vi "muPathSamplingFPGA28_SkipLiftScheme.vi"() -> ()   [LabVIEW 2017]
uses:
  <vilib>/rvi/Emulation/niFpgaSctlEmulationGetInTimedLoop.vi
  <vilib>/rvi/Emulation/niFpgaProcessEmulError.vi
  <vilib>/rvi/interface/RandomDataEmulation/niFpgaRandomDataHandleErrors.vi
  <vilib>/rvi/Emulation/niFpgaGetClockAttributes.vi
  <vilib>/rvi/Emulation/niFpgaEmulationReportErrorSimple.vi
  <vilib>/rvi/eio/common/nirviEmuTemplateMethod_errors.vi
  <vilib>/rvi/Emulation/niFpgaCriticalErrorInLSC.vi
  <vilib>/rvi/DataTransferAndStorage/Container/XNode/niFpgaContainer.xnode
  <vilib>/rvi/interface/RandomDataEmulation/nirviRandomDataFpgaReadWriteTemplate.vi
  <vilib>/eio/EIONode/EIONode.xnode
panel:
  out "direction_Next":u16
  out "y_image_Next":u16
  out "x_image_Next":u16
  out "Skip threshold":u16
  in  "pixel segment":u32
  out "x output":fxp<+/-,64,29>=0.00029289722442626953
  out "x sensor":fxp<+/-,20,5>
  out "y output":fxp<+/-,64,29>=0.29396580904722214
  out "y sensor":fxp<+/-,20,5>=-0.285125732421875
  in  "XY Clock (uSec)":fxp<+,32,32>=50.0
  out "z output":fxp<+/-,64,29>=-3.5890110712498426
  out "deflection sensor":fxp<+/-,20,5>=-0.271331787109375
  in  "Z Clock (uSec)":fxp<+,32,32>=10.0
  out "ToRead":u32
  in  "Stage Clock (uSec)":fxp<+,32,32>=500.0
  in  "Sampling Clock (uSec)":fxp<+,32,32>=1500.0
  in  "muPathUpdate Clock (uSec)":fxp<+,32,32>=2400.0
  out "zControlMode":bool
  out "a tor buffer":fxp<+,17,1>[](array[numeric])=[1.9999847412109375, 1.9999847412109375, 1.9999847412109375, 1.9999847412109375, 1.9999847412109375, 1.9999847412109375, 1.9999847412109375, 1.9999847412109375, 1.9999847412109375, 1.9999847412109375]
  out "b tor buffer":fxp<+,17,1>[](array[numeric])=[1.9999847412109375, 1.9999847412109375, 1.9999847412109375, 1.9999847412109375, 1.9999847412109375, 1.9999847412109375, 1.9999847412109375, 1.9999847412109375, 1.9999847412109375, 1.9999847412109375]
  out "x_pos":fxp<+/-,50,5>=0.005859375
  out "y_pos":fxp<+/-,50,5>=0.005859375
  out "signalToStop":bool
  in  "deflection control":T1={"SetPoint (V)"=0.0, "scanning I"=0.03125, "scanning P"=0.0498046875, "Initial I (V)"=0.0, "Upper Limit (V)"=8.0, "Lower Limit (V)"=-8.0, "approach I"=0.03125, "approach P"=0.0498046875}
  in  "z control":T2={"SetPoint (V)"=-0.19999980926513672, "I"=0.03125, "P"=0.0498046875, "Initial I (V)"=0.0, "Upper Limit (V)"=8.0, "Lower Limit (V)"=-8.0}
  out "stageIndicator":u8=1
  in  "x threshold":fxp<+/-,20,5>=0.0050048828125
  in  "y threshold":fxp<+/-,20,5>=0.0050048828125
  in  "z threshold":fxp<+/-,20,5>=0.0050048828125
  in  "deflection threshold":fxp<+/-,20,5>=0.0050048828125
  out "length":u16
  out "direction":u16
  out "x_FinalPos":fxp<+/-,50,5>
  out "y_FinalPos":fxp<+/-,50,5>
  out "SettleCheckBuffer":u16=25
  in  "y control":T3={"SetPoint (V)"=0.0, "scanning I"=0.03125, "scanning P"=0.0498046875, "Initial I (V)"=0.0, "Upper Limit (V)"=8.0, "Lower Limit (V)"=-8.0, "move I"=0.03125, "move P"=0.0302734375}
  in  "x control":T3={"SetPoint (V)"=0.0, "scanning I"=0.03125, "scanning P"=0.0498046875, "Initial I (V)"=0.0, "Upper Limit (V)"=8.0, "Lower Limit (V)"=-8.0, "move I"=0.03125, "move P"=0.0498046875}
  out "signalToInitialStageStop":bool
  out "mupathfinishSignal":bool
  in  "ImageToSample":T4={"image size_x"=256, "image size_y"=256, "sample start_x"=0.0, "sample start_y"=0.0, "sample end_x"=3.0, "sample end_y"=3.0}
  out "increment_x":fxp<+/-,50,5>=0.01171875
  out "increment_y":fxp<+/-,50,5>=0.01171875
  out "x_image_pos":u16
  out "y_image_pos":u16
  in  "x_scan threshold":fxp<+/-,20,5>=0.0050048828125
  in  "y_scan threshold":fxp<+/-,20,5>=0.0050048828125
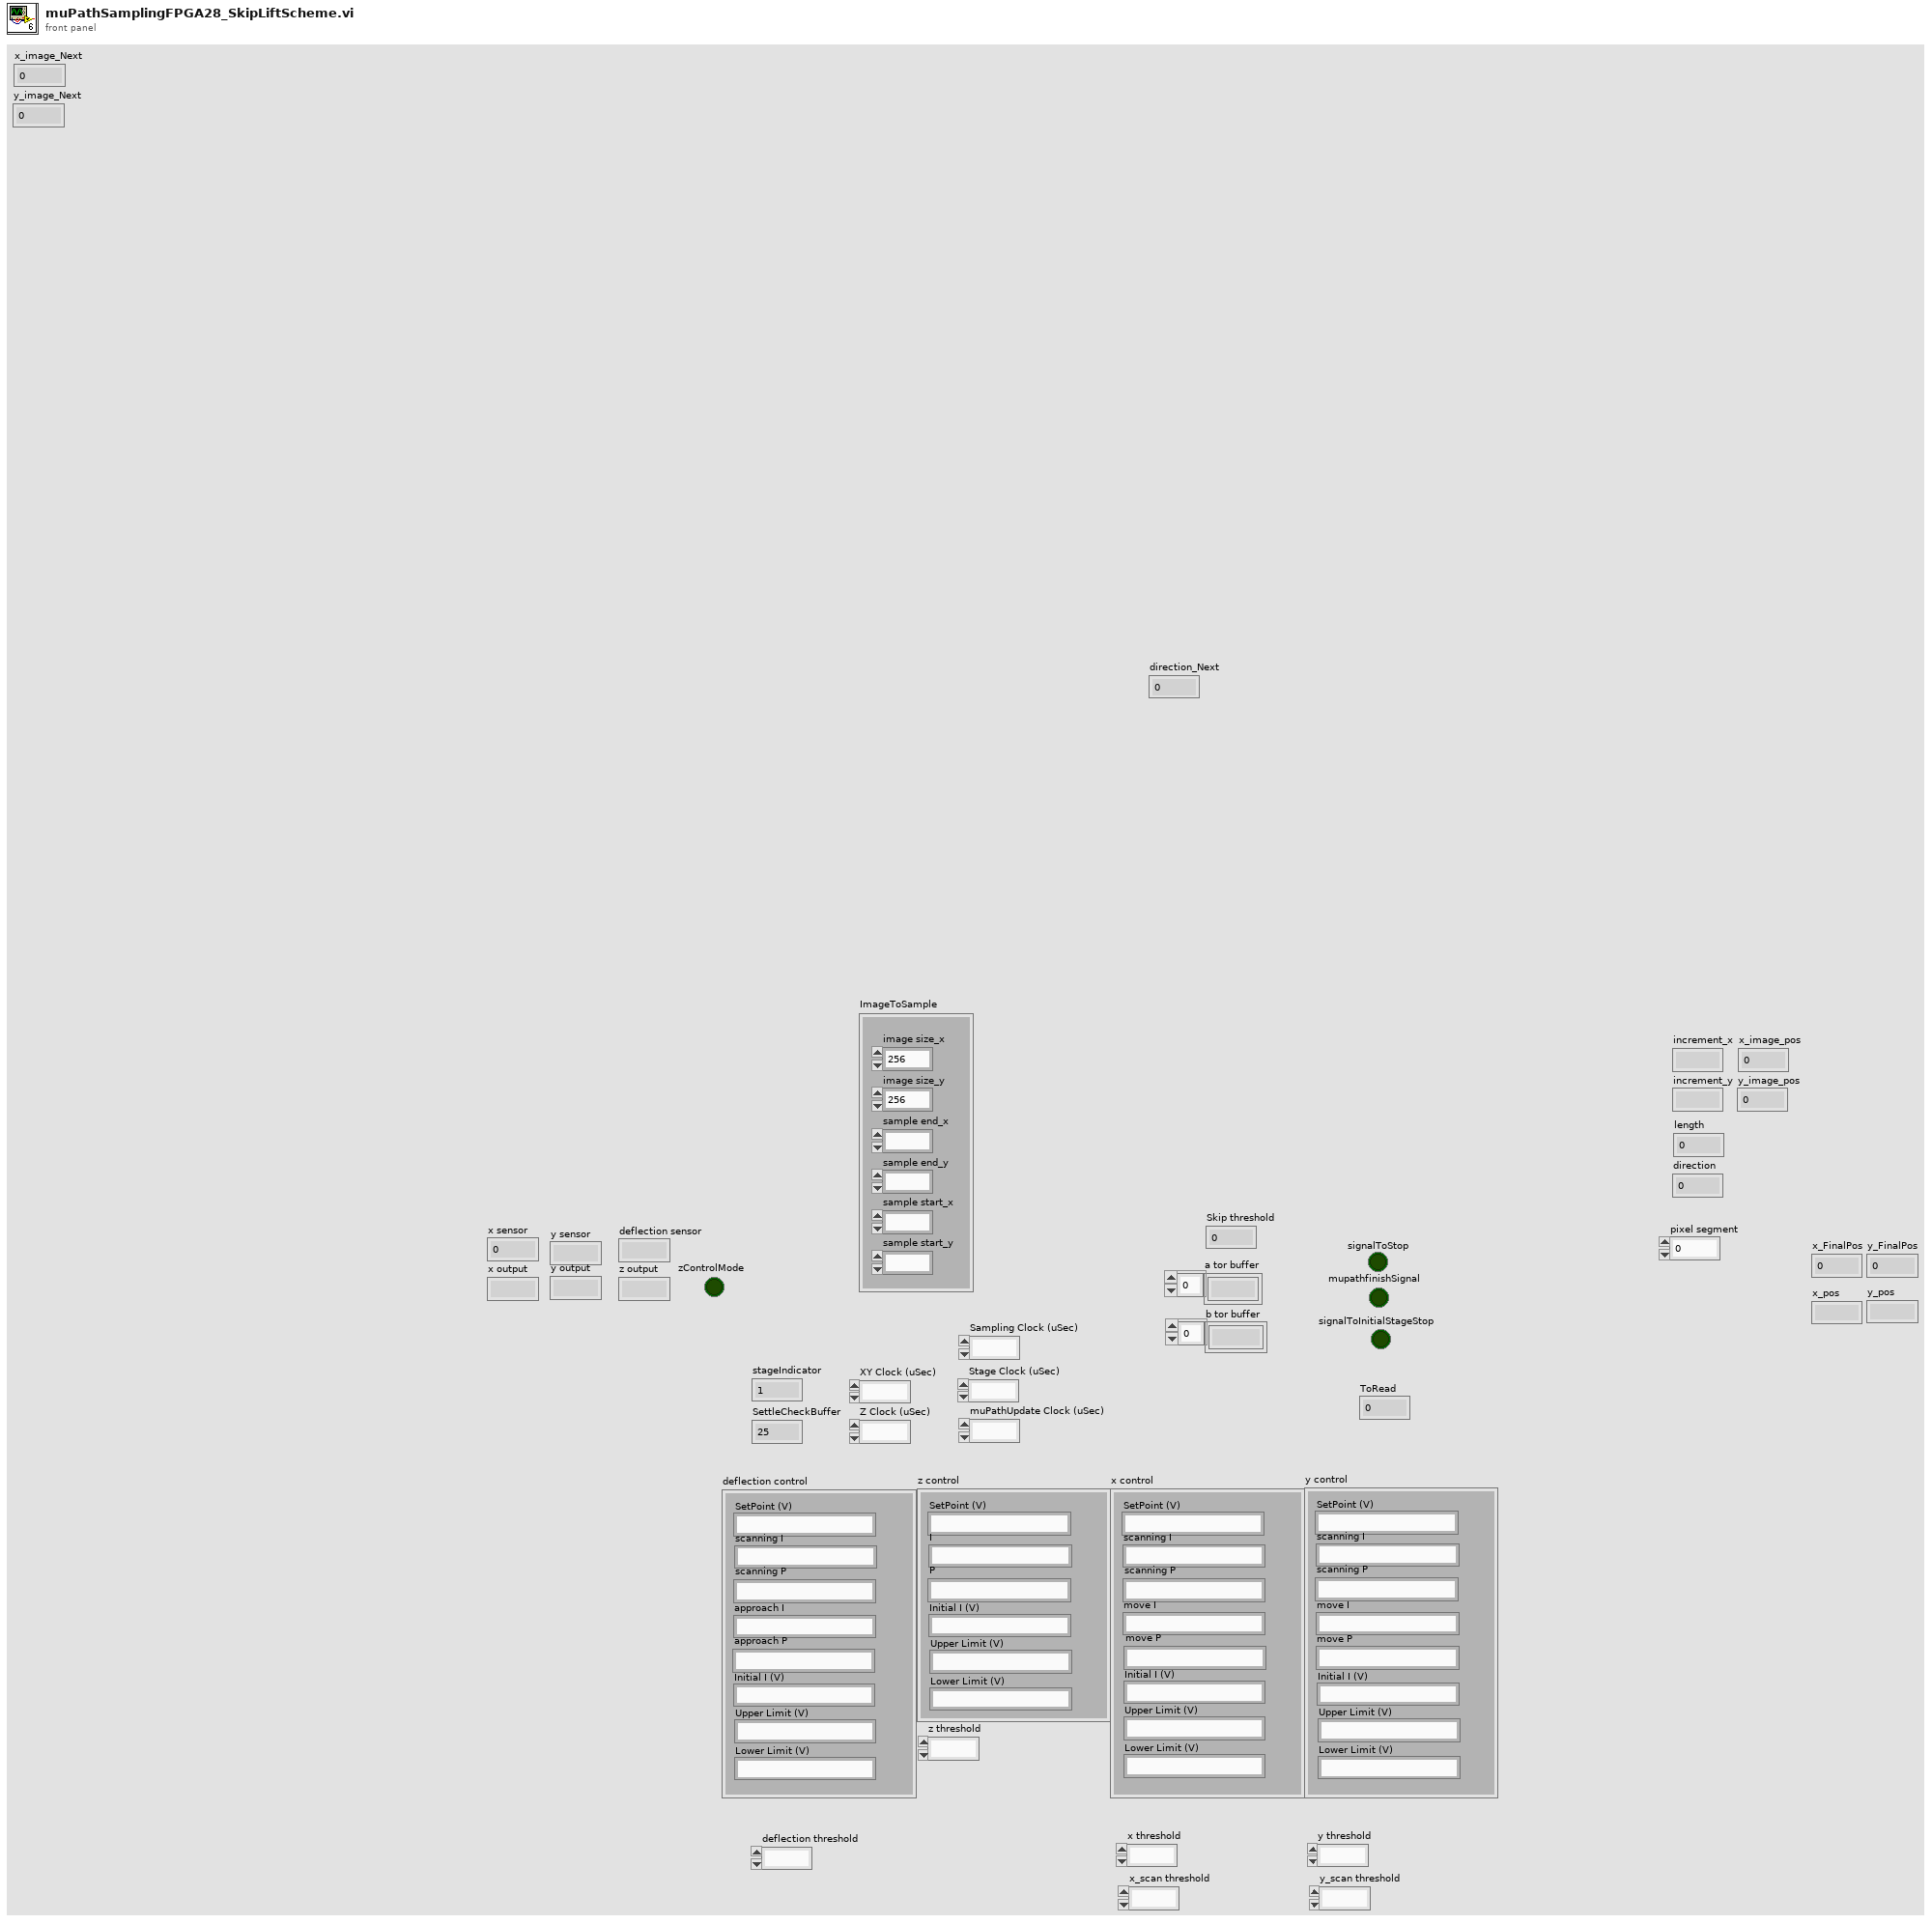
[diagram p1: front panel]
types:
  T1 = cluster{"SetPoint (V)":fxp<+/-,26,5>, "scanning I":fxp<+,21,13>, "scanning P":fxp<+,15,5>, "Initial I (V)":fxp<+/-,10,5>, "Upper Limit (V)":fxp<+/-,26,5>, "Lower Limit (V)":fxp<+/-,26,5>, "approach I":fxp<+,21,13>, "approach P":fxp<+,15,5>}
  T2 = cluster{"SetPoint (V)":fxp<+/-,26,5>, "I":fxp<+,21,13>, "P":fxp<+,15,5>, "Initial I (V)":fxp<+/-,10,5>, "Upper Limit (V)":fxp<+/-,26,5>, "Lower Limit (V)":fxp<+/-,26,5>}
  T3 = cluster{"SetPoint (V)":fxp<+/-,26,5>, "scanning I":fxp<+,21,13>, "scanning P":fxp<+,15,5>, "Initial I (V)":fxp<+/-,10,5>, "Upper Limit (V)":fxp<+/-,26,5>, "Lower Limit (V)":fxp<+/-,26,5>, "move I":fxp<+,21,13>, "move P":fxp<+,15,5>}
  T4 = cluster{"image size_x":u16, "image size_y":u16, "sample start_x":fxp<+/-,26,5>, "sample start_y":fxp<+/-,26,5>, "sample end_x":fxp<+/-,26,5>, "sample end_y":fxp<+/-,26,5>}
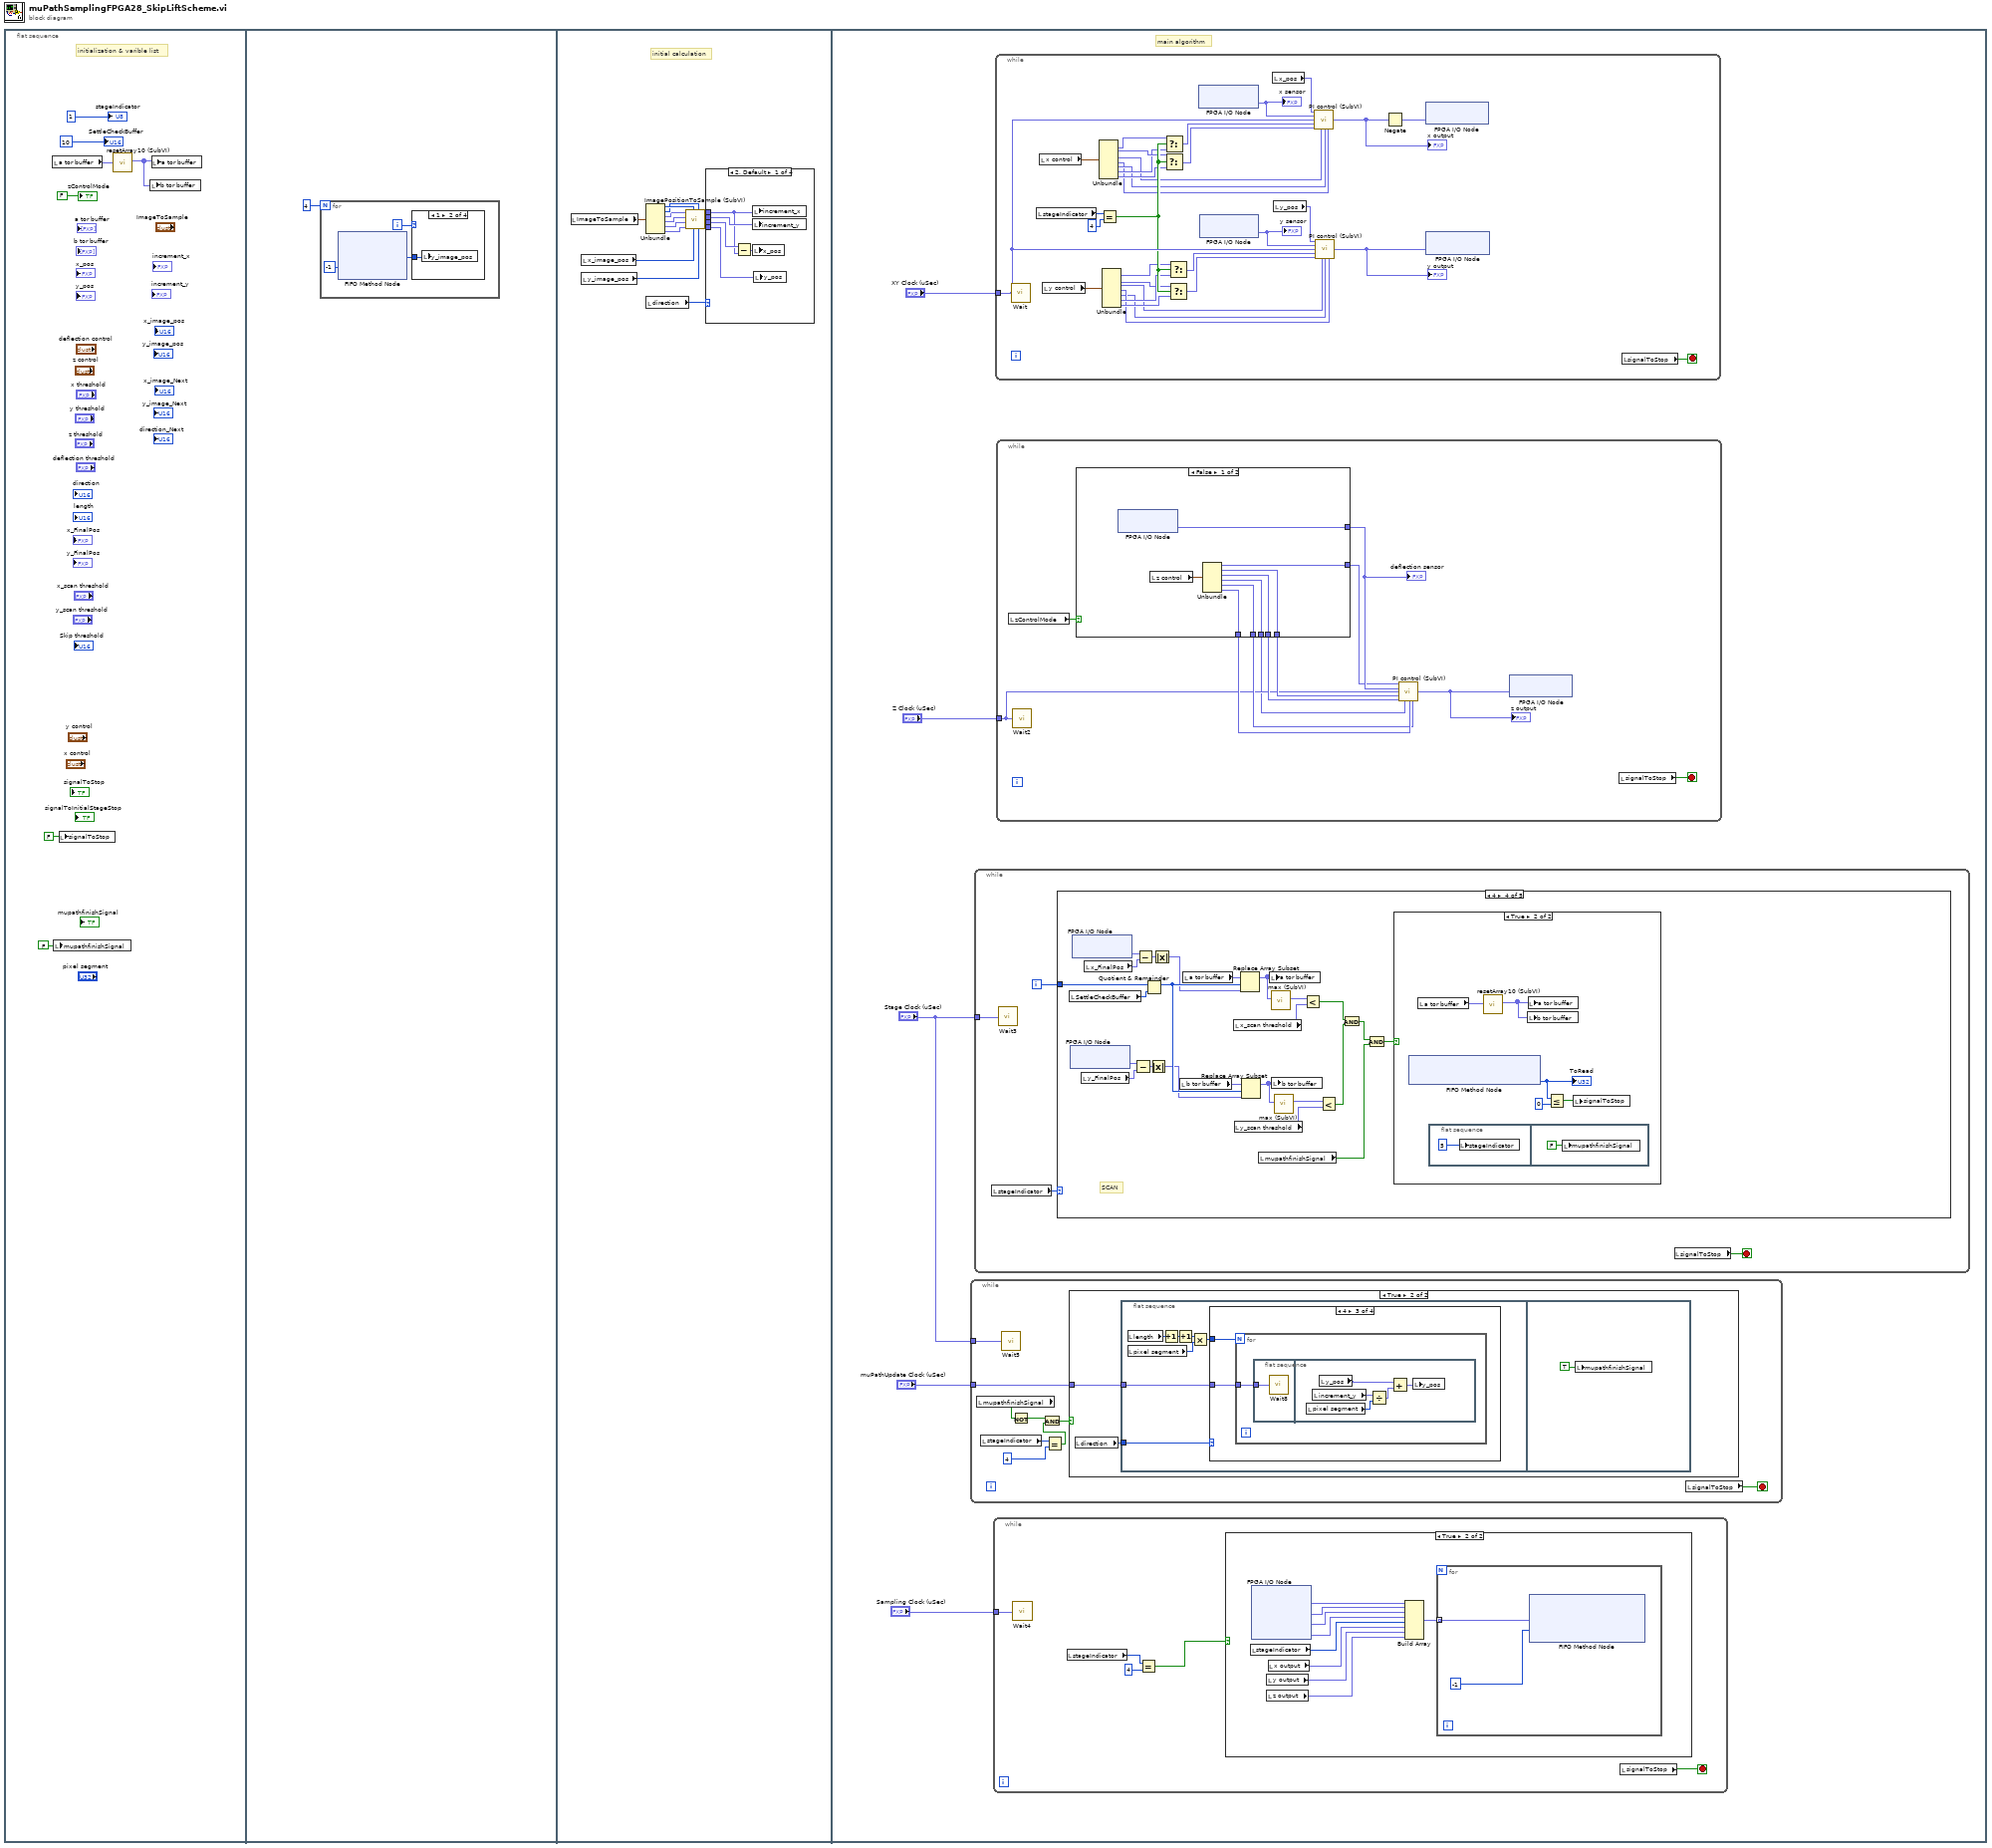
[diagram p0: block diagram]
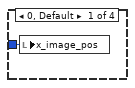
[diagram p2: hidden frame]
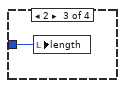
[diagram p3: hidden frame]
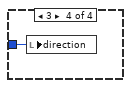
[diagram p4: hidden frame]
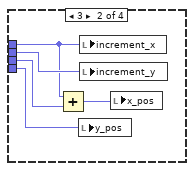
[diagram p5: hidden frame]
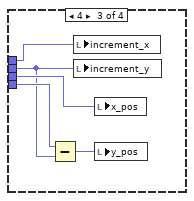
[diagram p6: hidden frame]
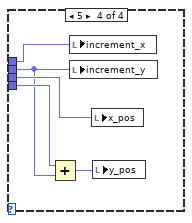
[diagram p7: hidden frame]
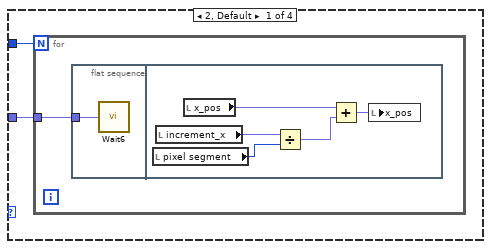
[diagram p9: hidden frame]
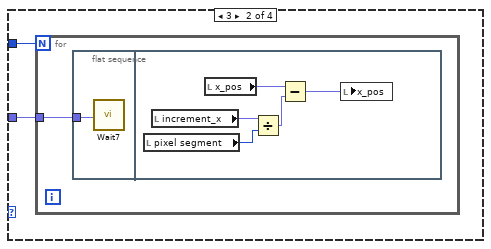
[diagram p10: hidden frame]
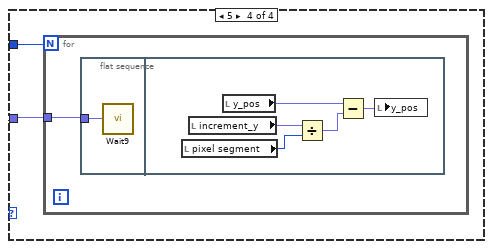
[diagram p11: hidden frame]
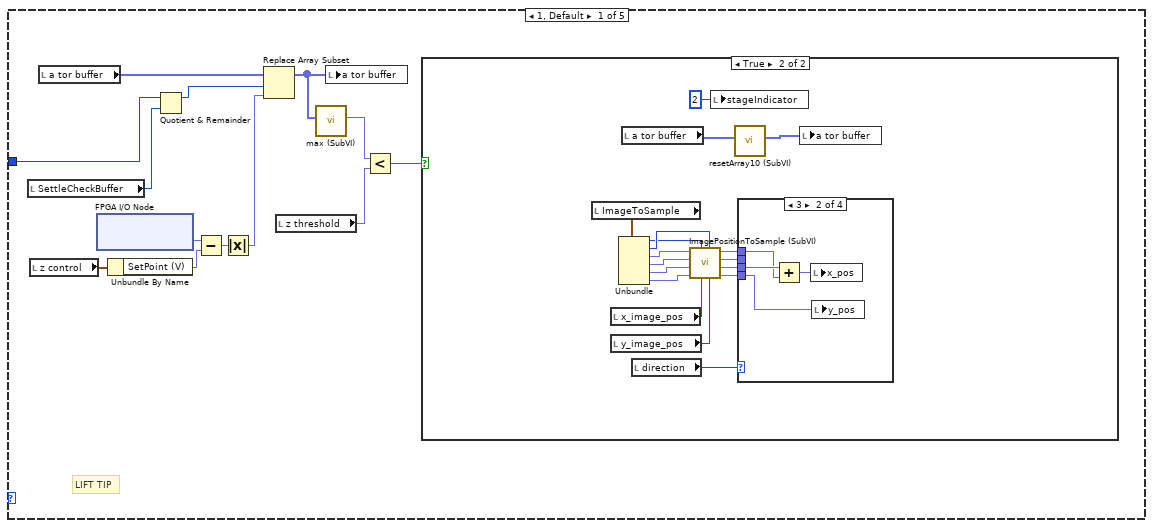
[diagram p13: hidden frame]
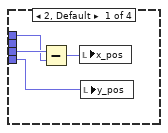
[diagram p15: hidden frame]
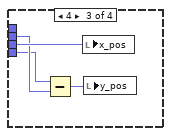
[diagram p16: hidden frame]
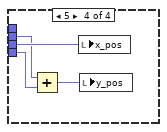
[diagram p17: hidden frame]
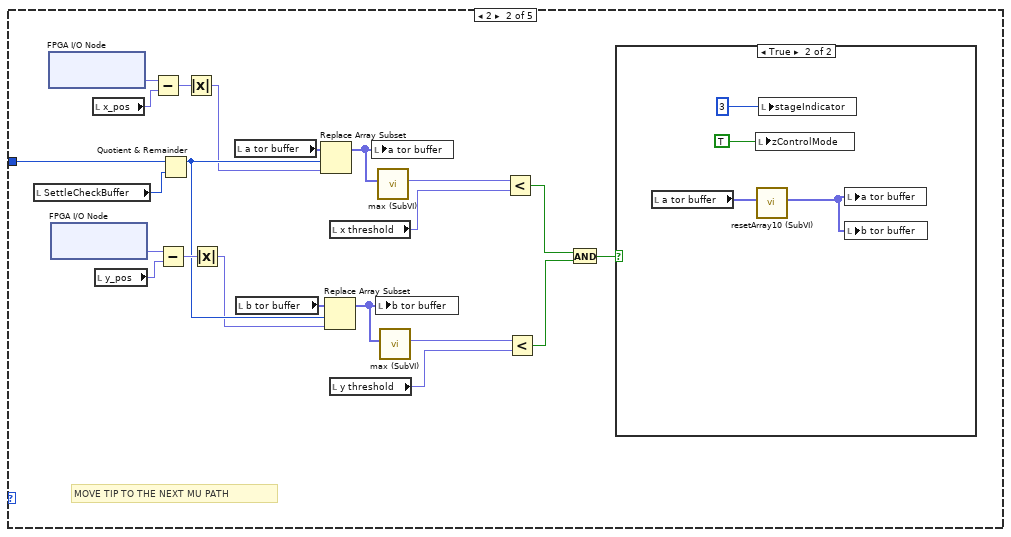
[diagram p18: hidden frame]
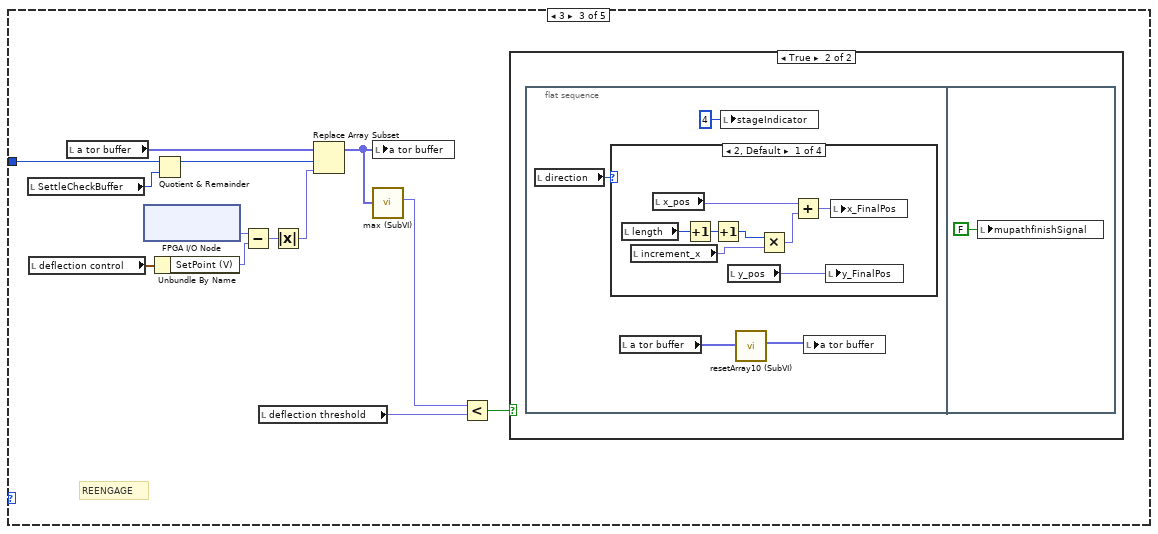
[diagram p20: hidden frame]
diagram:
  n1 = flat-sequence {
    frame #0 {
      # "initialization & varible list"
      n2 = local read "a tor buffer"() -> (w2:fxp<+,17,1>[])
      n3 = local write "mupathfinishSignal"(FALSE ("mupathfinishSignal")) -> ()
      n4 = local write "signalToStop"(FALSE ("signalToStop")) -> ()
      n5 = call "resetArray10 (SubVI).vi"("a samples in"=w2) -> ("a samples out"=w1:fxp<+/-,64,32>[])  [unwired: 10 in]
      n6 = local write "b tor buffer"(w1) -> ()
      n7 = local write "a tor buffer"(w1) -> ()
      "zControlMode" <- FALSE ("zControlMode")
      "stageIndicator" <- u8 1 ("stageIndicator")
      "SettleCheckBuffer" <- u16 10 ("SettleCheckLen")
    }
    frame #1 {
      n8 = for {
        N: 4 -> [_]
        i -> [w11]
        n9 = xnode ("FIFO Method Node")("Timeout"=-1) -> ("Element"=w9:u16)  [unwired: 1 in, 2 out]
        n10 = case shown="1" w11 {
          tunnel: w9 -> [w12 w13 w14 w15]
          frame 0, Default {
            n11 = local write "x_image_pos"(w12) -> ()
          }
          frame 1 {
            n12 = local write "y_image_pos"(w13) -> ()
          }
          frame 2 {
            n13 = local write "length"(w14) -> ()
          }
          frame 3 {
            n14 = local write "direction"(w15) -> ()
          }
        }
      }
    }
    frame #2 {
      # "initial calculation"
      n15 = local read "ImageToSample"() -> (w29:T4)
      n16 = local read "x_image_pos"() -> (w18:u16)
      n17 = local read "y_image_pos"() -> (w17:u16)
      n18 = Unbundle(w29) -> ("image size_x"=w28:u16, "image size_y"=w27:u16, "sample start_x"=w26:fxp<+/-,26,5>, "sample start_y"=w25:fxp<+/-,26,5>, "sample end_x"=w24:fxp<+/-,26,5>, "sample end_y"=w23:fxp<+/-,26,5>)
      n19 = local read "direction"() -> (w16:u16)
      n20 = call "ImagePositionToSample (SubVI).vi"("image_y"=w17, "image size_y"=w27, "image_x"=w18, "image size_x"=w28, "sample end_y"=w23, "sample end_x"=w24, "sample start_y"=w25, "sample start_x"=w26) -> ("sample_y"=w19:fxp<+/-,26,5>, "sample_x"=w20:fxp<+/-,26,5>, "increment_y"=w21:fxp<+/-,26,5>, "increment_x"=w22:fxp<+/-,26,5>)
      n21 = case shown="2, Default" w16 {
        tunnel: w22 -> [w32 w35 w44 w49]
        tunnel: w21 -> [w34 w39 w40 w45]
        tunnel: w20 -> [w33 w36 w42 w47]
        tunnel: w19 -> [w30 w38 w41 w46]
        frame 2, Default {
          n22 = Subtract(x=w33, y=w32) -> (x-y=w31:fxp<+/-,27,6>)
          n23 = local write "increment_y"(w34) -> ()
          n24 = local write "increment_x"(w32) -> ()
          n25 = local write "x_pos"(w31) -> ()
          n26 = local write "y_pos"(w30) -> ()
        }
        frame 3 {
          n27 = Add(x=w35, y=w36) -> (x+y=w37:fxp<+/-,27,6>)
          n28 = local write "y_pos"(w38) -> ()
          n29 = local write "increment_x"(w35) -> ()
          n30 = local write "increment_y"(w39) -> ()
          n31 = local write "x_pos"(w37) -> ()
        }
        frame 4 {
          n32 = Subtract(x=w41, y=w40) -> (x-y=w43:fxp<+/-,27,6>)
          n33 = local write "increment_x"(w44) -> ()
          n34 = local write "increment_y"(w40) -> ()
          n35 = local write "x_pos"(w42) -> ()
          n36 = local write "y_pos"(w43) -> ()
        }
        frame 5 {
          n37 = Add(x=w46, y=w45) -> (x+y=w48:fxp<+/-,27,6>)
          n38 = local write "increment_x"(w49) -> ()
          n39 = local write "increment_y"(w45) -> ()
          n40 = local write "x_pos"(w47) -> ()
          n41 = local write "y_pos"(w48) -> ()
        }
      }
    }
    frame #3 {
      # "main algorithm"
      n42 = while {
        tunnel: "Stage Clock (uSec)" -> [w62]
        tunnel: "muPathUpdate Clock (uSec)" -> [w59]
        stop <- w63 stop-if-true
        n43 = local read "mupathfinishSignal"() -> (w56:bool)
        n44 = local read "stageIndicator"() -> (w61:u8)
        n45 = call "Wait5"("Count(uSec)"=w62) -> ()  [unwired: 1 out]
        n46 = Not(x=w56) -> (.not. x?=w55:bool)
        n47 = Equal?(x=w61, y=u8 4) -> (x = y?=w58:bool)
        n48 = And(x=w55, y=w58) -> (x .and. y?=w57:bool)
        n49 = case shown="True" w57 {
          tunnel: w59 -> [_ w65]
          frame False {
          }
          frame True {
            n50 = local read "direction"() -> (w64:u16)
            n51 = flat-sequence {
              tunnel: w65 -> [w72]
              tunnel: w64 -> [w71]
              frame #0 {
                n52 = local read "length"() -> (w70:u16)
                n53 = local read "pixel segment"() -> (w68:u32)
                n54 = Increment(x=w70) -> (x+1=w67:u16)
                n55 = Increment(x=w67) -> (x+1=w66:u16)
                n56 = Multiply(x=w66, y=w68) -> (x*y=w69:u32)
                n57 = case shown="4" w71 {
                  tunnel: w72 -> [w74 w83 w92 w101]
                  tunnel: w69 -> [w73 w82 w91 w100]
                  frame 2, Default {
                    n58 = for {
                      N: w73 -> [_]
                      tunnel: w74 -> [w75]
                      n59 = flat-sequence {
                        tunnel: w75 -> [w76]
                        frame #0 {
                          n60 = call "Wait6"("Count(uSec)"=w76) -> ()  [unwired: 1 out]
                        }
                        frame #1 {
                          n61 = local read "pixel segment"() -> (w77:u32)
                          n62 = local read "increment_x"() -> (w79:fxp<+/-,50,5>)
                          n63 = local read "x_pos"() -> (w81:fxp<+/-,50,5>)
                          n64 = Divide(x=w79, y=w77) -> (x/y=w78:fxp<+/-,64,5>)
                          n65 = Add(x=w81, y=w78) -> (x+y=w80:fxp<+/-,64,6>)
                          n66 = local write "x_pos"(w80) -> ()
                        }
                      }
                    }
                  }
                  frame 3 {
                    n67 = for {
                      N: w82 -> [_]
                      tunnel: w83 -> [w84]
                      n68 = flat-sequence {
                        tunnel: w84 -> [w85]
                        frame #0 {
                          n69 = call "Wait7"("Count(uSec)"=w85) -> ()  [unwired: 1 out]
                        }
                        frame #1 {
                          n70 = local read "pixel segment"() -> (w86:u32)
                          n71 = local read "increment_x"() -> (w88:fxp<+/-,50,5>)
                          n72 = local read "x_pos"() -> (w90:fxp<+/-,50,5>)
                          n73 = Divide(x=w88, y=w86) -> (x/y=w87:fxp<+/-,64,5>)
                          n74 = Subtract(x=w90, y=w87) -> (x-y=w89:fxp<+/-,64,6>)
                          n75 = local write "x_pos"(w89) -> ()
                        }
                      }
                    }
                  }
                  frame 4 {
                    n76 = for {
                      N: w91 -> [_]
                      tunnel: w92 -> [w93]
                      n77 = flat-sequence {
                        tunnel: w93 -> [w94]
                        frame #0 {
                          n78 = call "Wait8"("Count(uSec)"=w94) -> ()  [unwired: 1 out]
                        }
                        frame #1 {
                          n79 = local read "pixel segment"() -> (w95:u32)
                          n80 = local read "increment_y"() -> (w97:fxp<+/-,50,5>)
                          n81 = local read "y_pos"() -> (w99:fxp<+/-,50,5>)
                          n82 = Divide(x=w97, y=w95) -> (x/y=w96:fxp<+/-,64,5>)
                          n83 = Add(x=w99, y=w96) -> (x+y=w98:fxp<+/-,64,6>)
                          n84 = local write "y_pos"(w98) -> ()
                        }
                      }
                    }
                  }
                  frame 5 {
                    n85 = for {
                      N: w100 -> [_]
                      tunnel: w101 -> [w102]
                      n86 = flat-sequence {
                        tunnel: w102 -> [w103]
                        frame #0 {
                          n87 = call "Wait9"("Count(uSec)"=w103) -> ()  [unwired: 1 out]
                        }
                        frame #1 {
                          n88 = local read "pixel segment"() -> (w105:u32)
                          n89 = local read "increment_y"() -> (w106:fxp<+/-,50,5>)
                          n90 = local read "y_pos"() -> (w108:fxp<+/-,50,5>)
                          n91 = Divide(x=w106, y=w105) -> (x/y=w104:fxp<+/-,64,5>)
                          n92 = Subtract(x=w108, y=w104) -> (x-y=w107:fxp<+/-,64,6>)
                          n93 = local write "y_pos"(w107) -> ()
                        }
                      }
                    }
                  }
                }
              }
              frame #1 {
                n94 = local write "mupathfinishSignal"(TRUE ("mupathfinishSignal")) -> ()
              }
            }
          }
        }
        n95 = local read "signalToStop"() -> (w63:bool)
      }
      n96 = while {
        tunnel: "Stage Clock (uSec)" -> [w127]
        i -> [w126]
        stop <- w129 stop-if-true
        n97 = local read "stageIndicator"() -> (w128:u8)
        n98 = call "Wait3"("Count(uSec)"=w127) -> ()  [unwired: 1 out]
        n99 = case shown="4" w128 {
          tunnel: w126 -> [w141 w190 w210 w269 _]
          frame 1, Default {
            # "LIFT TIP"
            n100 = local read "SettleCheckBuffer"() -> (w140:u16)
            n101 = local read "z control"() -> (w136:T2)
            n102 = local read "a tor buffer"() -> (w139:fxp<+,17,1>[])
            n103 = xnode "FPGA I/O Node"() -> ("Mod1/AI2"=w137:fxp<+/-,20,5>)  [unwired: 1 in, 1 out]
            n104 = Unbundle By Name(w136) -> ("SetPoint (V)"=w135:fxp<+/-,26,5>)
            n105 = Quotient & Remainder(x=w141, y=w140) -> (x-y*floor(x/y)=w134:i32)  [unwired: 1 out]
            n106 = Subtract(x=w137, y=w135) -> (x-y=w138:fxp<+/-,27,6>)
            n107 = Absolute Value(x=w138) -> (abs(x)=w133:fxp<+,26,5>)
            n108 = Replace Array Subset(array=w139, new element=w133, index=w134) -> (w131:fxp<+,17,1>[])
            n109 = local read "z threshold"() -> (w132:fxp<+/-,20,5>)
            n110 = call "max (SubVI).vi"("initialized array"=w131) -> ("y"=w130:fxp<+/-,64,32>)  [unwired: 10 in]
            n111 = local write "a tor buffer"(w131) -> ()
            n112 = Less?(x=w130, y=w132) -> (x < y?=w142:bool)
            n113 = case shown="True" w142 {
              frame False {
              }
              frame True {
                n114 = local read "ImageToSample"() -> (w145:T4)
                n115 = local read "x_image_pos"() -> (w152:u16)
                n116 = local read "y_image_pos"() -> (w153:u16)
                n117 = Unbundle(w145) -> ("image size_x"=w146:u16, "image size_y"=w147:u16, "sample start_x"=w148:fxp<+/-,26,5>, "sample start_y"=w149:fxp<+/-,26,5>, "sample end_x"=w150:fxp<+/-,26,5>, "sample end_y"=w151:fxp<+/-,26,5>)
                n118 = local read "a tor buffer"() -> (w143:fxp<+,17,1>[])
                n119 = local read "direction"() -> (w154:u16)
                n120 = call "ImagePositionToSample (SubVI).vi"("image_y"=w153, "image size_y"=w147, "image_x"=w152, "image size_x"=w146, "sample end_y"=w151, "sample end_x"=w150, "sample start_y"=w149, "sample start_x"=w148) -> ("sample_y"=w155:fxp<+/-,26,5>, "sample_x"=w156:fxp<+/-,26,5>, "increment_y"=w158:fxp<+/-,26,5>, "increment_x"=w157:fxp<+/-,26,5>)
                n121 = local write "stageIndicator"(u8 2 ("stageIndicator")) -> ()
                n122 = call "resetArray10 (SubVI).vi"("a samples in"=w143) -> ("a samples out"=w144:fxp<+/-,64,32>[])  [unwired: 10 in]
                n123 = case shown="3" w154 {
                  tunnel: w155 -> [w163 w167 w168 w173]
                  tunnel: w156 -> [w162 w166 w171 w175]
                  tunnel: w157 -> [w161 w165 _ _]
                  tunnel: w158 -> [_ _ w169 w174]
                  frame 2, Default {
                    n124 = Subtract(x=w162, y=w161) -> (x-y=w160:fxp<+/-,27,6>)
                    n125 = local write "x_pos"(w160) -> ()
                    n126 = local write "y_pos"(w163) -> ()
                  }
                  frame 3 {
                    n127 = Add(x=w166, y=w165) -> (x+y=w164:fxp<+/-,27,6>)
                    n128 = local write "x_pos"(w164) -> ()
                    n129 = local write "y_pos"(w167) -> ()
                  }
                  frame 4 {
                    n130 = Subtract(x=w168, y=w169) -> (x-y=w170:fxp<+/-,27,6>)
                    n131 = local write "x_pos"(w171) -> ()
                    n132 = local write "y_pos"(w170) -> ()
                  }
                  frame 5 {
                    n133 = Add(x=w174, y=w173) -> (x+y=w172:fxp<+/-,27,6>)
                    n134 = local write "x_pos"(w175) -> ()
                    n135 = local write "y_pos"(w172) -> ()
                  }
                }
                n136 = local write "a tor buffer"(w144) -> ()
              }
            }
          }
          frame 2 {
            # "MOVE TIP TO THE NEXT MU PATH"
            n137 = local read "SettleCheckBuffer"() -> (w189:u16)
            n138 = xnode "FPGA I/O Node"() -> ("Mod1/AI0"=w196:fxp<+/-,20,5>)  [unwired: 1 in, 1 out]
            n139 = xnode "FPGA I/O Node"() -> ("Mod1/AI1"=w194:fxp<+/-,20,5>)  [unwired: 1 in, 1 out]
            n140 = local read "x_pos"() -> (w193:fxp<+/-,50,5>)
            n141 = local read "y_pos"() -> (w192:fxp<+/-,50,5>)
            n142 = Subtract(x=w196, y=w193) -> (x-y=w197:fxp<+/-,51,6>)
            n143 = Subtract(x=w194, y=w192) -> (x-y=w195:fxp<+/-,51,6>)
            n144 = Quotient & Remainder(x=w190, y=w189) -> (x-y*floor(x/y)=w187:i32)  [unwired: 1 out]
            n145 = Absolute Value(x=w197) -> (abs(x)=w185:fxp<+,50,5>)
            n146 = Absolute Value(x=w195) -> (abs(x)=w184:fxp<+,50,5>)
            n147 = local read "a tor buffer"() -> (w188:fxp<+,17,1>[])
            n148 = local read "b tor buffer"() -> (w186:fxp<+,17,1>[])
            n149 = Replace Array Subset(array=w188, new element=w185, index=w187) -> (w178:fxp<+,17,1>[])
            n150 = Replace Array Subset(array=w186, new element=w184, index=w187) -> (w176:fxp<+,17,1>[])
            n151 = local read "x threshold"() -> (w183:fxp<+/-,20,5>)
            n152 = local read "y threshold"() -> (w182:fxp<+/-,20,5>)
            n153 = local write "a tor buffer"(w178) -> ()
            n154 = local write "b tor buffer"(w176) -> ()
            n155 = call "max (SubVI).vi"("initialized array"=w178) -> ("y"=w179:fxp<+/-,64,32>)  [unwired: 10 in]
            n156 = call "max (SubVI).vi"("initialized array"=w176) -> ("y"=w177:fxp<+/-,64,32>)  [unwired: 10 in]
            n157 = Less?(x=w179, y=w183) -> (x < y?=w181:bool)
            n158 = Less?(x=w177, y=w182) -> (x < y?=w180:bool)
            n159 = And(x=w181, y=w180) -> (x .and. y?=w191:bool)
            n160 = case shown="True" w191 {
              frame False {
              }
              frame True {
                n161 = local read "a tor buffer"() -> (w199:fxp<+,17,1>[])
                n162 = local write "zControlMode"(TRUE ("signalToStop")) -> ()
                n163 = call "resetArray10 (SubVI).vi"("a samples in"=w199) -> ("a samples out"=w198:fxp<+/-,64,32>[])  [unwired: 10 in]
                n164 = local write "stageIndicator"(u8 3 ("stageIndicator")) -> ()
                n165 = local write "a tor buffer"(w198) -> ()
                n166 = local write "b tor buffer"(w198) -> ()
              }
            }
          }
          frame 3 {
            # "REENGAGE"
            n167 = local read "SettleCheckBuffer"() -> (w209:u16)
            n168 = local read "deflection control"() -> (w212:T1)
            n169 = local read "a tor buffer"() -> (w207:fxp<+,17,1>[])
            n170 = xnode "FPGA I/O Node"() -> ("Mod1/AI3"=w213:fxp<+/-,20,5>)  [unwired: 1 in, 1 out]
            n171 = Quotient & Remainder(x=w210, y=w209) -> (x-y*floor(x/y)=w208:i32)  [unwired: 1 out]
            n172 = Unbundle By Name(w212) -> ("SetPoint (V)"=w211:fxp<+/-,26,5>)
            n173 = Subtract(x=w213, y=w211) -> (x-y=w214:fxp<+/-,27,6>)
            n174 = local read "deflection threshold"() -> (w204:fxp<+/-,20,5>)
            n175 = Absolute Value(x=w214) -> (abs(x)=w206:fxp<+,26,5>)
            n176 = Replace Array Subset(array=w207, new element=w206, index=w208) -> (w203:fxp<+,17,1>[])
            n177 = local write "a tor buffer"(w203) -> ()
            n178 = call "max (SubVI).vi"("initialized array"=w203) -> ("y"=w202:fxp<+/-,64,32>)  [unwired: 10 in]
            n179 = Less?(x=w202, y=w204) -> (x < y?=w205:bool)
            n180 = case shown="True" w205 {
              frame False {
              }
              frame True {
                n181 = flat-sequence {
                  frame #0 {
                    n182 = local read "direction"() -> (w217:u16)
                    n183 = case shown="2, Default" w217 {
                      frame 2, Default {
                        n184 = local read "length"() -> (w219:u16)
                        n185 = local read "increment_x"() -> (w224:fxp<+/-,50,5>)
                        n186 = local read "x_pos"() -> (w226:fxp<+/-,50,5>)
                        n187 = Increment(x=w219) -> (x+1=w220:u16)
                        n188 = Increment(x=w220) -> (x+1=w221:u16)
                        n189 = local read "y_pos"() -> (w222:fxp<+/-,50,5>)
                        n190 = Multiply(x=w221, y=w224) -> (x*y=w223:fxp<+/-,64,21>)
                        n191 = Add(x=w226, y=w223) -> (x+y=w225:fxp<+/-,64,22>)
                        n192 = local write "y_FinalPos"(w222) -> ()
                        n193 = local write "x_FinalPos"(w225) -> ()
                      }
                      frame 3 {
                        n194 = local read "length"() -> (w229:u16)
                        n195 = local read "increment_x"() -> (w232:fxp<+/-,50,5>)
                        n196 = local read "x_pos"() -> (w234:fxp<+/-,50,5>)
                        n197 = Increment(x=w229) -> (x+1=w228:u16)
                        n198 = Increment(x=w228) -> (x+1=w227:u16)
                        n199 = Multiply(x=w227, y=w232) -> (x*y=w231:fxp<+/-,64,21>)
                        n200 = local read "y_pos"() -> (w230:fxp<+/-,50,5>)
                        n201 = Subtract(x=w234, y=w231) -> (x-y=w233:fxp<+/-,64,22>)
                        n202 = local write "y_FinalPos"(w230) -> ()
                        n203 = local write "x_FinalPos"(w233) -> ()
                      }
                      frame 4 {
                        n204 = local read "length"() -> (w237:u16)
                        n205 = local read "increment_y"() -> (w240:fxp<+/-,50,5>)
                        n206 = local read "y_pos"() -> (w242:fxp<+/-,50,5>)
                        n207 = Increment(x=w237) -> (x+1=w236:u16)
                        n208 = Increment(x=w236) -> (x+1=w235:u16)
                        n209 = Multiply(x=w235, y=w240) -> (x*y=w239:fxp<+/-,64,21>)
                        n210 = local read "x_pos"() -> (w238:fxp<+/-,50,5>)
                        n211 = Add(x=w242, y=w239) -> (x+y=w241:fxp<+/-,64,22>)
                        n212 = local write "y_FinalPos"(w241) -> ()
                        n213 = local write "x_FinalPos"(w238) -> ()
                      }
                      frame 5 {
                        n214 = local read "increment_y"() -> (w247:fxp<+/-,50,5>)
                        n215 = local read "length"() -> (w245:u16)
                        n216 = local read "y_pos"() -> (w250:fxp<+/-,50,5>)
                        n217 = Increment(x=w245) -> (x+1=w244:u16)
                        n218 = Increment(x=w244) -> (x+1=w243:u16)
                        n219 = Multiply(x=w243, y=w247) -> (x*y=w248:fxp<+/-,64,21>)
                        n220 = local read "x_pos"() -> (w246:fxp<+/-,50,5>)
                        n221 = Subtract(x=w250, y=w248) -> (x-y=w249:fxp<+/-,64,22>)
                        n222 = local write "y_FinalPos"(w249) -> ()
                        n223 = local write "x_FinalPos"(w246) -> ()
                      }
                    }
                    n224 = local read "a tor buffer"() -> (w216:fxp<+,17,1>[])
                    n225 = local write "stageIndicator"(u8 4 ("stageIndicator")) -> ()
                    n226 = call "resetArray10 (SubVI).vi"("a samples in"=w216) -> ("a samples out"=w215:fxp<+/-,64,32>[])  [unwired: 10 in]
                    n227 = local write "a tor buffer"(w215) -> ()
                  }
                  frame #1 {
                    n228 = local write "mupathfinishSignal"(FALSE ("mupathfinishSignal")) -> ()
                  }
                }
              }
            }
          }
          frame 4 {
            # "SCAN"
            n229 = local read "SettleCheckBuffer"() -> (w268:u16)
            n230 = xnode "FPGA I/O Node"() -> ("Mod1/AI1"=w273:fxp<+/-,20,5>)  [unwired: 1 in, 1 out]
            n231 = xnode "FPGA I/O Node"() -> ("Mod1/AI0"=w275:fxp<+/-,20,5>)  [unwired: 1 in, 1 out]
            n232 = local read "y_FinalPos"() -> (w270:fxp<+/-,50,5>)
            n233 = local read "x_FinalPos"() -> (w271:fxp<+/-,50,5>)
            n234 = Subtract(x=w273, y=w270) -> (x-y=w272:fxp<+/-,51,6>)
            n235 = Subtract(x=w275, y=w271) -> (x-y=w274:fxp<+/-,51,6>)
            n236 = Quotient & Remainder(x=w269, y=w268) -> (x-y*floor(x/y)=w267:i32)  [unwired: 1 out]
            n237 = Absolute Value(x=w272) -> (abs(x)=w266:fxp<+,50,5>)
            n238 = Absolute Value(x=w274) -> (abs(x)=w265:fxp<+,50,5>)
            n239 = local read "b tor buffer"() -> (w263:fxp<+,17,1>[])
            n240 = local read "a tor buffer"() -> (w264:fxp<+,17,1>[])
            n241 = local read "x_scan threshold"() -> (w262:fxp<+/-,20,5>)
            n242 = local read "y_scan threshold"() -> (w261:fxp<+/-,20,5>)
            n243 = Replace Array Subset(array=w264, new element=w265, index=w267) -> (w255:fxp<+,17,1>[])
            n244 = Replace Array Subset(array=w263, new element=w266, index=w267) -> (w258:fxp<+,17,1>[])
            n245 = local read "mupathfinishSignal"() -> (w252:bool)
            n246 = local write "a tor buffer"(w255) -> ()
            n247 = call "max (SubVI).vi"("initialized array"=w255) -> ("y"=w256:fxp<+/-,64,32>)  [unwired: 10 in]
            n248 = local write "b tor buffer"(w258) -> ()
            n249 = call "max (SubVI).vi"("initialized array"=w258) -> ("y"=w257:fxp<+/-,64,32>)  [unwired: 10 in]
            n250 = Less?(x=w256, y=w262) -> (x < y?=w260:bool)
            n251 = Less?(x=w257, y=w261) -> (x < y?=w259:bool)
            n252 = And(x=w260, y=w259) -> (x .and. y?=w253:bool)
            n253 = And(x=w253, y=w252) -> (x .and. y?=w254:bool)
            n254 = case shown="True" w254 {
              frame False {
              }
              frame True {
                n255 = xnode ("FIFO Method Node")() -> ("Number of Elements to Read"=w280:u32)  [unwired: 1 in, 1 out]
                "ToRead" <- w280
                n256 = local read "a tor buffer"() -> (w277:fxp<+,17,1>[])
                n257 = flat-sequence {
                  frame #0 {
                    n258 = local write "stageIndicator"(u8 5 ("stageIndicator")) -> ()
                  }
                  frame #1 {
                    n259 = local write "mupathfinishSignal"(FALSE ("mupathfinishSignal")) -> ()
                  }
                }
                n260 = call "resetArray10 (SubVI).vi"("a samples in"=w277) -> ("a samples out"=w276:fxp<+/-,64,32>[])  [unwired: 10 in]
                n261 = local write "b tor buffer"(w276) -> ()
                n262 = local write "a tor buffer"(w276) -> ()
                n263 = Less Or Equal?(x=w280, y=u32 0) -> (x <= y?=w278:bool)
                n264 = local write "signalToStop"(w278) -> ()
              }
            }
          }
          frame 5 {
            n265 = flat-sequence {
              frame #0 {
                n266 = for {
                  N: 4 -> [_]
                  i -> [w286]
                  n267 = xnode ("FIFO Method Node")("Timeout"=-1) -> ("Element"=w284:u16)  [unwired: 1 in, 2 out]
                  n268 = case shown="0, Default" w286 {
                    tunnel: w284 -> [w287 w288 w289 w290]
                    frame 0, Default {
                      n269 = local write "x_image_Next"(w287) -> ()
                    }
                    frame 1 {
                      n270 = local write "y_image_Next"(w288) -> ()
                    }
                    frame 2 {
                      n271 = local write "length"(w289) -> ()
                    }
                    frame 3 {
                      n272 = local write "direction_Next"(w290) -> ()
                    }
                  }
                }
              }
              frame #1 {
                n273 = local read "direction_Next"() -> (w315:u16)
                n274 = case shown="2, Default" w315 {
                  tunnel: [w360 w364 w367 w368] -> w307
                  tunnel: [w359 w362 w365 w370] -> w306
                  frame 2, Default {
                    n275 = local read "x_image_Next"() -> (w361:u16)
                    n276 = local read "y_image_Next"() -> (w359:u16)
                    n277 = Decrement(x=w361) -> (x-1=w360:u16)
                  }
                  frame 3 {
                    n278 = local read "y_image_Next"() -> (w362:u16)
                    n279 = local read "x_image_Next"() -> (w363:u16)
                    n280 = Increment(x=w363) -> (x+1=w364:u16)
                  }
                  frame 4 {
                    n281 = local read "y_image_Next"() -> (w366:u16)
                    n282 = local read "x_image_Next"() -> (w367:u16)
                    n283 = Decrement(x=w366) -> (x-1=w365:u16)
                  }
                  frame 5 {
                    n284 = local read "x_image_Next"() -> (w368:u16)
                    n285 = local read "y_image_Next"() -> (w369:u16)
                    n286 = Increment(x=w369) -> (x+1=w370:u16)
                  }
                }
                n287 = local read "x_FinalPos"() -> (w297:fxp<+/-,50,5>)
                n288 = local read "y_FinalPos"() -> (w296:fxp<+/-,50,5>)
                n289 = local read "ImageToSample"() -> (w310:T4)
                n290 = Unbundle(w310) -> ("image size_x"=w314:u16, "image size_y"=w308:u16, "sample start_x"=w313:fxp<+/-,26,5>, "sample start_y"=w312:fxp<+/-,26,5>, "sample end_x"=w311:fxp<+/-,26,5>, "sample end_y"=w309:fxp<+/-,26,5>)
                n291 = call "ImagePositionToSample (SubVI).vi"("image_y"=w306, "image size_y"=w308, "image_x"=w307, "image size_x"=w314, "sample end_y"=w309, "sample end_x"=w311, "sample start_y"=w312, "sample start_x"=w313) -> ("sample_y"=w298:fxp<+/-,26,5>, "sample_x"=w299:fxp<+/-,26,5>, "increment_y"=w294:fxp<+/-,26,5>)  [unwired: 1 out]
                n292 = local read "Skip threshold"() -> (w295:u16)
                n293 = Subtract(x=w299, y=w297) -> (x-y=w302:fxp<+/-,51,6>)
                n294 = Subtract(x=w298, y=w296) -> (x-y=w301:fxp<+/-,51,6>)
                n295 = Square(x=w302) -> (x^2=w304:fxp<+,64,10>)
                n296 = Square(x=w301) -> (x^2=w305:fxp<+,64,10>)
                n297 = Add(x=w304, y=w305) -> (x+y=w303:fxp<+,64,11>)
                n298 = Multiply(x=w295, y=w294) -> (x*y=w293:fxp<+/-,42,21>)
                n299 = Square Root(x=w303) -> (sqrt(x)=w300:fxp<+,64,6>)
                n300 = Round Toward +Infinity(x=w300) -> (ceil(x): smallest int >= x=w292:fxp<+,7,7>)
                n301 = Greater Or Equal?(x=w293, y=w292) -> (x >= y?=w291:bool)
                n302 = case shown="False" w291 {
                  frame False {
                    # "NOT SKIP - LIFT"
                    n303 = local read "direction_Next"() -> (w317:u16)
                    n304 = local read "x_image_Next"() -> (w319:u16)
                    n305 = local read "y_image_Next"() -> (w318:u16)
                    n306 = local write "stageIndicator"(u8 1 ("stageIndicator")) -> ()
                    n307 = local write "zControlMode"(FALSE ("zControlMode")) -> ()
                    n308 = local write "x_image_pos"(w319) -> ()
                    n309 = local write "y_image_pos"(w318) -> ()
                    n310 = local write "direction"(w317) -> ()
                  }
                  frame True {
                    # "SKIP - NOT LIFT"
                    n311 = flat-sequence {
                      frame #0 {
                        n312 = local read "direction_Next"() -> (w324:u16)
                        n313 = local read "y_image_Next"() -> (w323:u16)
                        n314 = local write "y_image_pos"(w323) -> ()
                        n315 = local read "x_image_Next"() -> (w322:u16)
                        n316 = local write "x_image_pos"(w322) -> ()
                        n317 = local write "direction"(w324) -> ()
                      }
                      frame #1 {
                        n318 = local read "ImageToSample"() -> (w325:T4)
                        n319 = local read "x_image_pos"() -> (w336:u16)
                        n320 = local read "y_image_pos"() -> (w337:u16)
                        n321 = Unbundle(w325) -> ("image size_x"=w326:u16, "image size_y"=w327:u16, "sample start_x"=w328:fxp<+/-,26,5>, "sample start_y"=w329:fxp<+/-,26,5>, "sample end_x"=w330:fxp<+/-,26,5>, "sample end_y"=w331:fxp<+/-,26,5>)
                        n322 = local read "direction"() -> (w338:u16)
                        n323 = call "ImagePositionToSample (SubVI).vi"("image_y"=w337, "image size_y"=w327, "image_x"=w336, "image size_x"=w326, "sample end_y"=w331, "sample end_x"=w330, "sample start_y"=w329, "sample start_x"=w328) -> ("sample_y"=w335:fxp<+/-,26,5>, "sample_x"=w334:fxp<+/-,26,5>, "increment_y"=w333:fxp<+/-,26,5>, "increment_x"=w332:fxp<+/-,26,5>)
                        n324 = case shown="2, Default" w338 {
                          tunnel: w332 -> [w341 w344 w353 w358]
                          tunnel: w333 -> [w343 w348 w349 w354]
                          tunnel: w334 -> [w342 w345 w351 w356]
                          tunnel: w335 -> [w339 w347 w350 w355]
                          frame 2, Default {
                            n325 = Subtract(x=w342, y=w341) -> (x-y=w340:fxp<+/-,27,6>)
                            n326 = local write "increment_y"(w343) -> ()
                            n327 = local write "increment_x"(w341) -> ()
                            n328 = local write "x_pos"(w340) -> ()
                            n329 = local write "y_pos"(w339) -> ()
                          }
                          frame 3 {
                            n330 = Add(x=w344, y=w345) -> (x+y=w346:fxp<+/-,27,6>)
                            n331 = local write "y_pos"(w347) -> ()
                            n332 = local write "increment_x"(w344) -> ()
                            n333 = local write "increment_y"(w348) -> ()
                            n334 = local write "x_pos"(w346) -> ()
                          }
                          frame 4 {
                            n335 = Subtract(x=w350, y=w349) -> (x-y=w352:fxp<+/-,27,6>)
                            n336 = local write "increment_x"(w353) -> ()
                            n337 = local write "increment_y"(w349) -> ()
                            n338 = local write "x_pos"(w351) -> ()
                            n339 = local write "y_pos"(w352) -> ()
                          }
                          frame 5 {
                            n340 = Add(x=w355, y=w354) -> (x+y=w357:fxp<+/-,27,6>)
                            n341 = local write "increment_x"(w358) -> ()
                            n342 = local write "increment_y"(w354) -> ()
                            n343 = local write "x_pos"(w356) -> ()
                            n344 = local write "y_pos"(w357) -> ()
                          }
                        }
                      }
                    }
                    n345 = local write "stageIndicator"(u8 2 ("stageIndicator")) -> ()
                  }
                }
              }
            }
          }
        }
        n346 = local read "signalToStop"() -> (w129:bool)
      }
      n347 = while {
        tunnel: "Sampling Clock (uSec)" -> [w114]
        stop <- w113 stop-if-true
        n348 = call "Wait4"("Count(uSec)"=w114) -> ()  [unwired: 1 out]
        n349 = local read "stageIndicator"() -> (w111:u8)
        n350 = Equal?(x=w111, y=u8 4) -> (x = y?=w112:bool)
        n351 = case shown="True" w112 {
          frame False {
          }
          frame True {
            n352 = local read "stageIndicator"() -> (w118:u8)
            n353 = xnode "FPGA I/O Node"() -> ("Mod1/AI0"=w122:fxp<+/-,20,5>, "Mod1/AI1"=w121:fxp<+/-,20,5>, "Mod1/AI2"=w120:fxp<+/-,20,5>, "Mod1/AI3"=w119:fxp<+/-,20,5>)  [unwired: 4 in, 4 out]
            n354 = local read "y output"() -> (w116:fxp<+/-,64,29>)
            n355 = local read "z output"() -> (w115:fxp<+/-,64,29>)
            n356 = local read "x output"() -> (w117:fxp<+/-,64,29>)
            n357 = Build Array(w122, w121, w120, w119, w118, w117, w116, w115) -> (w123:fxp<+/-,64,29>[])
            n358 = for {
              tunnel: w123 -> [w124] mode=indexing
              n359 = xnode ("FIFO Method Node")("Element"=w124, "Timeout"=-1) -> ()  [unwired: 1 in, 2 out]
            }
          }
        }
        n360 = local read "signalToStop"() -> (w113:bool)
      }
      n361 = while {
        tunnel: "XY Clock (uSec)" -> [w435]
        stop <- w432 stop-if-true
        n362 = call "Wait"("Count(uSec)"=w435) -> ()  [unwired: 1 out]
        n363 = local read "stageIndicator"() -> (w427:u8)
        n364 = local read "x control"() -> (w429:T3)
        n365 = local read "y control"() -> (w428:T3)
        n366 = Unbundle(w429) -> ("scanning I"=w424:fxp<+,21,13>, "scanning P"=w423:fxp<+,15,5>, "Initial I (V)"=w418:fxp<+/-,10,5>, "Upper Limit (V)"=w416:fxp<+/-,26,5>, "Lower Limit (V)"=w417:fxp<+/-,26,5>, "move I"=w422:fxp<+,21,13>, "move P"=w421:fxp<+,15,5>)  [unwired: 1 out]
        n367 = Equal?(x=w427, y=u8 4) -> (x = y?=w425:bool)
        n368 = Unbundle(w428) -> ("scanning I"=w413:fxp<+,21,13>, "scanning P"=w412:fxp<+,15,5>, "Initial I (V)"=w411:fxp<+/-,10,5>, "Upper Limit (V)"=w410:fxp<+/-,26,5>, "Lower Limit (V)"=w409:fxp<+/-,26,5>, "move I"=w415:fxp<+,21,13>, "move P"=w414:fxp<+,15,5>)  [unwired: 1 out]
        n369 = Select(t=w424, s=w425, f=w422) -> (s? t:f=w420:fxp<+,21,13>)
        n370 = Select(t=w423, s=w425, f=w421) -> (s? t:f=w419:fxp<+,15,5>)
        n371 = Select(t=w413, s=w425, f=w415) -> (s? t:f=w408:fxp<+,21,13>)
        n372 = Select(t=w412, s=w425, f=w414) -> (s? t:f=w407:fxp<+,15,5>)
        n373 = xnode "FPGA I/O Node"() -> ("Mod1/AI0"=w436:fxp<+/-,20,5>)  [unwired: 1 in, 1 out]
        "x sensor" <- w436
        n374 = xnode "FPGA I/O Node"() -> ("Mod1/AI1"=w438:fxp<+/-,20,5>)  [unwired: 1 in, 1 out]
        "y sensor" <- w438
        n375 = local read "x_pos"() -> (w433:fxp<+/-,50,5>)
        n376 = local read "y_pos"() -> (w434:fxp<+/-,50,5>)
        n377 = call "PI control (SubVI).vi"("SetPoint"=w433, "Feedback"=w436, "Clock"=w435, "I"=w420, "P"=w419, "Initial I"=w418, "Lower Limit"=w417, "Upper Limit in"=w416) -> ("Output"=w431:fxp<+/-,20,5>)  [unwired: 7 in]
        "x output" <- w431
        n378 = call "PI control (SubVI).vi"("SetPoint"=w434, "Feedback"=w438, "Clock"=w435, "I"=w408, "P"=w407, "Initial I"=w411, "Lower Limit"=w409, "Upper Limit in"=w410) -> ("Output"=w437:fxp<+/-,20,5>)  [unwired: 7 in]
        "y output" <- w437
        n379 = Negate(x=w431) -> (-x=w430:fxp<+/-,21,6>)
        n380 = xnode "FPGA I/O Node"("Mod8/AO0"=w430) -> ()  [unwired: 1 in, 1 out]
        n381 = xnode "FPGA I/O Node"("Mod8/AO1"=w437) -> ()  [unwired: 1 in, 1 out]
        n382 = local read "signalToStop"() -> (w432:bool)
      }
      n383 = while {
        tunnel: "Z Clock (uSec)" -> [w372]
        stop <- w380 stop-if-true
        n384 = local read "zControlMode"() -> (w379:bool)
        n385 = call "Wait2"("Count(uSec)"=w372) -> ()  [unwired: 1 out]
        n386 = case shown="False" w379 {
          tunnel: [w388 w405] -> w378
          tunnel: [w387 w402] -> w377
          tunnel: [w383 w393] -> w376
          tunnel: [w384 w390] -> w375
          tunnel: [w386 w401] -> w374
          tunnel: [w385 w400] -> w373
          tunnel: [w382 w399] -> w371
          frame False {
            n387 = xnode "FPGA I/O Node"() -> ("Mod1/AI2"=w388:fxp<+/-,20,5>)  [unwired: 1 in, 1 out]
            n388 = local read "z control"() -> (w389:T2)
            n389 = Unbundle(w389) -> ("SetPoint (V)"=w387:fxp<+/-,26,5>, "I"=w383:fxp<+,21,13>, "P"=w384:fxp<+,15,5>, "Initial I (V)"=w382:fxp<+/-,10,5>, "Upper Limit (V)"=w385:fxp<+/-,26,5>, "Lower Limit (V)"=w386:fxp<+/-,26,5>)
          }
          frame True {
            n390 = local read "deflection control"() -> (w404:T1)
            n391 = local read "stageIndicator"() -> (w398:u8)
            n392 = xnode "FPGA I/O Node"() -> ("Mod1/AI3"=w406:fxp<+/-,20,5>)  [unwired: 1 in, 1 out]
            n393 = Equal?(x=w398, y=u8 4) -> (x = y?=w396:bool)
            n394 = Unbundle(w404) -> ("SetPoint (V)"=w403:fxp<+/-,26,5>, "scanning I"=w395:fxp<+,21,13>, "scanning P"=w392:fxp<+,15,5>, "Initial I (V)"=w399:fxp<+/-,10,5>, "Upper Limit (V)"=w400:fxp<+/-,26,5>, "Lower Limit (V)"=w401:fxp<+/-,26,5>, "approach I"=w394:fxp<+,21,13>, "approach P"=w391:fxp<+,15,5>)
            n395 = Negate(x=w406) -> (-x=w405:fxp<+/-,21,6>)
            n396 = Select(t=w395, s=w396, f=w394) -> (s? t:f=w393:fxp<+,21,13>)
            n397 = Select(t=w392, s=w396, f=w391) -> (s? t:f=w390:fxp<+,15,5>)
            n398 = Negate(x=w403) -> (-x=w402:fxp<+/-,27,6>)
          }
        }
        "deflection sensor" <- w378
        n399 = call "PI control (SubVI).vi"("SetPoint"=w377, "Feedback"=w378, "Clock"=w372, "I"=w376, "P"=w375, "Initial I"=w371, "Lower Limit"=w374, "Upper Limit in"=w373) -> ("Output"=w381:fxp<+/-,20,5>)  [unwired: 7 in]
        "z output" <- w381
        n400 = xnode "FPGA I/O Node"("Mod8/AO2"=w381) -> ()  [unwired: 1 in, 1 out]
        n401 = local read "signalToStop"() -> (w380:bool)
      }
    }
  }
